vi "Fetch Multi Eval Meas List ES Flatness MinR Results.vi"(7 "Result Type (Current)":i32(ring) items=["Current", "Average", "Extreme", "Standard Deviation"], 8 "error in (no error)":errorcluster, 9 "Range (1)":T1=1, 10 "Instance (1)":T2=1, 11 "VISA resource name":refnum<visa-resource-name>) -> (0 "error out":errorcluster, 1 "ES Flatness MinR Results":dbl[](array[numeric]) format="%^.3e", 2 "Reliability":i32, 3 "VISA resource name out":refnum<visa-resource-name>)   [LabVIEW 2020, in "Rohde&Schwarz CMXP NR FR2 Measurement.lvlib"]
doc: "Returns equalizer spectrum flatness single value results (minimum within a range) for all measured list mode segments.\n\nAttributes:\nRSCMXPNRFR2M_ATTR_FETCH_MULTI_EVAL_MEASUREMENT_LIST_ESF_MINR_AVERAGE_RESULTS\nRSCMXPNRFR2M_ATTR_FETCH_MULTI_EVAL_MEASUREMENT_LIST_ESF_MINR_CURRENT_RESULTS\nRSCMXPNRFR2M_ATTR_FETCH_MULTI_EVAL_MEASUREMENT_LIST_ESF_MINR_EXTREME_RESULTS\nRSCMXPNRFR2M_ATTR_FETCH_MULTI_EVAL_MEASUREMENT_LIST_ESF_MINR_STANDARD_DEVIATION_RESULTS\n\nRemote-control commands:\nFETCh:NRMMw:MEAS<i>:MEValuation:LIST:ESFLatness:MINR<no>:AVERage?\nFETCh:NRMMw:MEAS<i>:MEValuation:LIST:ESFLatness:MINR<no>:CURRent?\nFETCh:NRMMw:MEAS<i>:MEValuation:LIST:ESFLatness:MINR<no>:EXTReme?\nFETCh:NRMMw:MEAS<i>:MEValuation:LIST:ESFLatness:MINR<no>:SDEViation?"
uses:
  <instrlib>/Rohde&Schwarz CMXP NR FR2 Measurement/Rohde&Schwarz CMXP NR FR2 Measurement.lvlib
  <instrlib>/Rohde&Schwarz CMXP NR FR2 Measurement/Private/_Instance.ctl
  <instrlib>/Rohde&Schwarz CMXP NR FR2 Measurement/Private/_Range.ctl
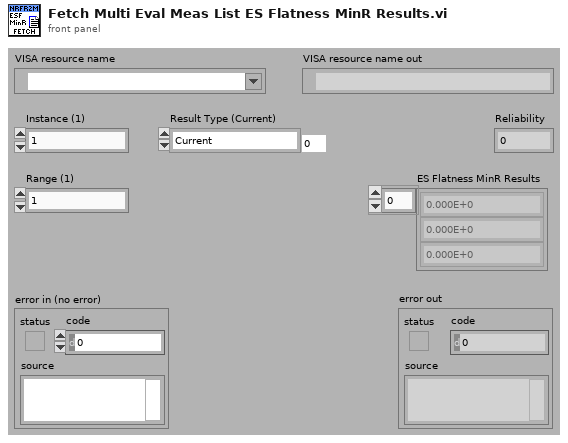
[diagram p1: front panel]
types:
  T1 = typedef "Rohde&Schwarz CMXP NR FR2 Measurement.lvlib/_Range.ctl" = i32
  T2 = typedef "Rohde&Schwarz CMXP NR FR2 Measurement.lvlib/_Instance.ctl" = i32
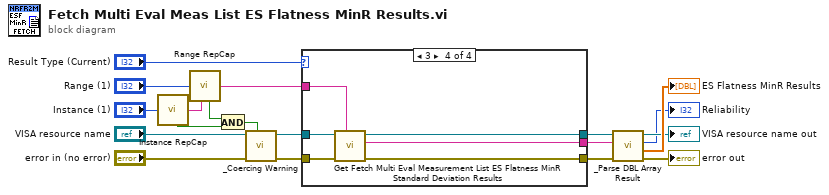
[diagram p0: block diagram]
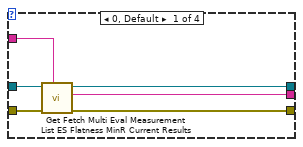
[diagram p2: hidden frame]
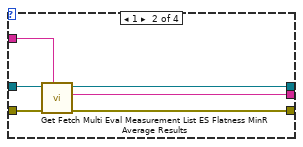
[diagram p3: hidden frame]
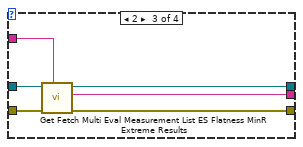
[diagram p4: hidden frame]
diagram:
  n1 = call <instrlib>:"Instance RepCap.vi"("Instance In"="Instance (1)") -> ("In Range?"=w17:bool, "RepCap Identifier Out"=w1:string)  [unwired: 1 in]
  n2 = call <instrlib>:"Range RepCap.vi"("Range In"="Range (1)", "RepCap String In (\"\")"=w1) -> ("In Range?"=w19:bool, "RepCap Identifier Out"=w13:string)
  n3 = And(x=w19, y=w17) -> (x .and. y?=w18:bool)
  n4 = call <instrlib>:"_Coercing Warning.vi"("In Range?"=w18, "error in (no error)"="error in (no error)", "VISA resource name"="VISA resource name") -> ("error out"=w11:errorcluster, "VISA resource name out"=w12:refnum<visa-resource-name>)  [unwired: 7 in]
  n5 = case shown="3" "Result Type (Current)" {
    tunnel: w13 -> [w25 w31 w37 w43]
    tunnel: w12 -> [w24 w30 w36 w42]
    tunnel: w11 -> [w23 w29 w35 w41]
    tunnel: [w22 w28 w34 w40] -> w8
    tunnel: [w21 w27 w33 w39] -> w9
    tunnel: [w20 w26 w32 w38] -> w10
    frame 0, Default {
      n6 = call "Get Fetch Multi Eval Measurement List ES Flatness MinR Current Results"("Repeated Capabilities"=w25, "error in (no error)"=w23, "instrument handle"=w24) -> ("error out"=w22:errorcluster, "Fetch Multi Eval Measurement List ES Flatness MinR Current Results"=w21:string, "instrument handle out"=w20:refnum<visa-resource-name>)  [unwired: 6 in]
    }
    frame 1 {
      n7 = call "Get Fetch Multi Eval Measurement List ES Flatness MinR Average Results"("Repeated Capabilities"=w31, "error in (no error)"=w29, "instrument handle"=w30) -> ("error out"=w28:errorcluster, "Fetch Multi Eval Measurement List ES Flatness MinR Average Results"=w27:string, "instrument handle out"=w26:refnum<visa-resource-name>)  [unwired: 6 in]
    }
    frame 2 {
      n8 = call "Get Fetch Multi Eval Measurement List ES Flatness MinR Extreme Results"("Repeated Capabilities"=w37, "error in (no error)"=w35, "instrument handle"=w36) -> ("error out"=w34:errorcluster, "Fetch Multi Eval Measurement List ES Flatness MinR Extreme Results"=w33:string, "instrument handle out"=w32:refnum<visa-resource-name>)  [unwired: 6 in]
    }
    frame 3 {
      n9 = call "Get Fetch Multi Eval Measurement List ES Flatness MinR Standard Deviation Results"("Repeated Capabilities"=w43, "error in (no error)"=w41, "instrument handle"=w42) -> ("error out"=w40:errorcluster, "Fetch Multi Eval Measurement List ES Flatness MinR Standard Deviation Results"=w39:string, "instrument handle out"=w38:refnum<visa-resource-name>)  [unwired: 6 in]
    }
  }
  n10 = call <instrlib>:"_Parse DBL Array Result.vi"("error in (no error)"=w8, "Input String"=w9, "VISA resource name"=w10) -> ("error out"=→"error out":errorcluster, "Results"=→"ES Flatness MinR Results":dbl[], "Reliability"=→"Reliability":i32, "VISA resource name out"=→"VISA resource name out":refnum<visa-resource-name>)  [unwired: 5 in]
